vi "Enumerate Step Types.vi"(8 "error in (no error)":errorcluster, 11 "Search Directory":path) -> (0 "error out":errorcluster, 3 "Step Names":string[](array[string]))   [LabVIEW 2015, in "Configuration Tool.lvlib"]
uses:
  Configuration Tool.lvlib
  <vilib>/Utility/error.llb/Error Cluster From Error Code.vi
  <vilib>/ErrorRing/Error Ring.xnode
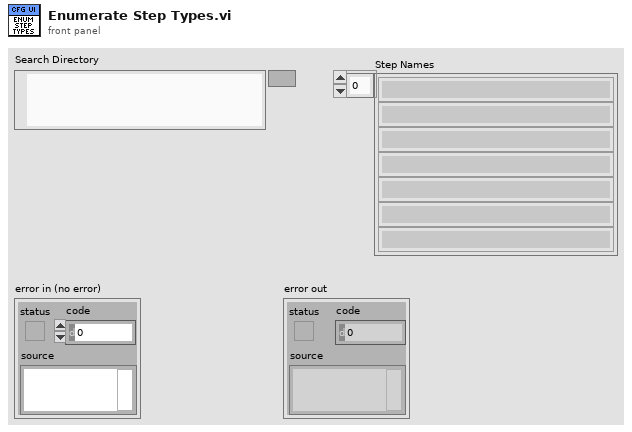
[diagram p1: front panel]
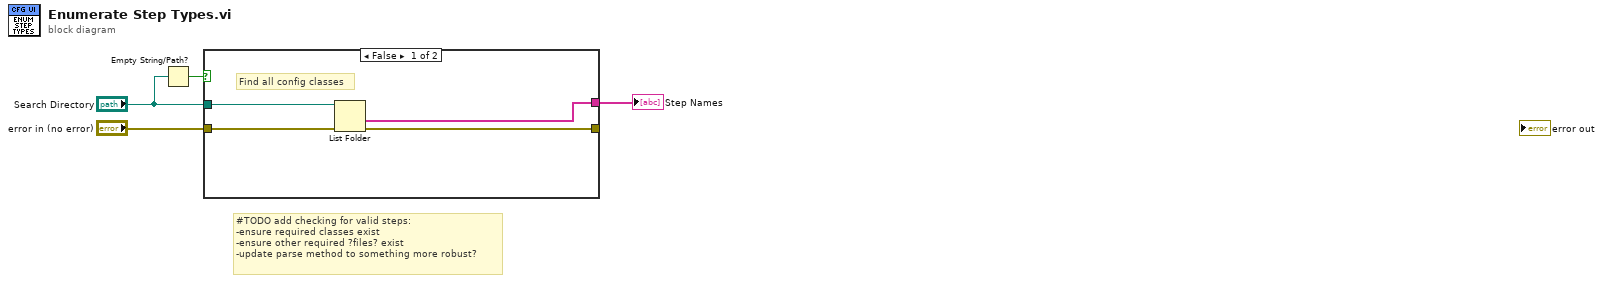
[diagram p0: block diagram]
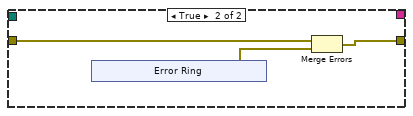
[diagram p2: hidden frame]
diagram:
  # "#TODO add checking for valid steps:\n-ensure required classes exist\n-ensure other required ?files? exist\n-update parse method to something more robust?"
  n1 = Empty String/Path?(string/path="Search Directory") -> (empty?=w2:bool)
  n2 = case shown="False" w2 {
    tunnel: "error in (no error)" -> [w8 w11]
    tunnel: "Search Directory" -> [w7 _]
    tunnel: [w6 w10] -> _
    tunnel: [w5 _] -> w1
    frame False {
      # "Find all config classes"
      n3 = List Folder(path=w7, error in=w8) -> (folder names=w5:string[], error out=w6:errorcluster)  [unwired: 2 in, 2 out]
    }
    frame True {
      n4 = xnode "Error Ring"() -> ("error out"=w9:errorcluster)
      n5 = Merge Errors(w11, w9) -> (w10:errorcluster)
    }
  }
  "Step Names" <- w1
